vi "General Error Handler CORE.vi"(0 "[error code] (0)":i32 caption="[Fehlercode] (0)" format="%0.0f", 1 "[user-defined codes]":i32[](array[numeric]) caption="[Benutzerspezif. Codes]", 2 "[user-defined descriptions]":string[](array[string]) caption="[Benutzerspezif. Beschreibungen]", 5 "[error source] (\" \")":string caption="[Fehlerquelle] (\" \")", 7 "String to Format (not a refnum)":refnum<vi> caption="String nach Format (kein Refnum)", 9 "type of dialog (OK msg:1)":T2=enum."OK message" caption="Dialog-Typ (OK msg:1)", 11 "error in (no error)":errorcluster caption="Fehler (Eingang, kein Fehler)", 12 "[exception action] (none:0)":i32(ring) caption="[Ausnahmeaktion] (none:0)" items=["Keine Ausnahme", "Bei Übereinstimmung Fehler ignorieren", "bei Übereinstimmung Fehler ausgeben"], 13 "[exception code]":i32 caption="[Ausnahmecode]" format="%0.0f", 14 "[exception source]":string caption="[Ausnahmequelle]") -> (3 "stop event propagated":bool caption="Stopereignis propagieren", 4 "error?":bool caption="Fehler?", 6 "code out":i32 caption="Code (Ausgabe)" format="%0.0f", 8 "source out":string caption="Quelle (Ausgang)", 10 "message":string=" INSTRUKTIONEN:\r\rAllgemeine Nutzung:  Bei der Benutzung von SubVIs, die die Fehler(Eingang)-/Fehler(Ausgang)- (oder Fehler-I/O-) Struktur verwenden, plazieren Sie diesen Handler dort, wo Sie den Benutzer auf aufgetretene Fehler hinweisen wollen, typischerweise geschieht dies am Ende eines I/O-Datenpfades als letzte Aktion des Programms.  Wenn der Fehlerstatus einen Fehler angibt, erzeugt der Handler eine Nachricht, die den Fehler und dessen Ursprung beschreibt.  Ist Dialogtyp = 1 (Voreinstellung), wird die Fehlermeldung angezeigt und der Benutzer kann diese lediglich bestätigen.  Ist Dialogtyp = 2, kann der Benutzer die Meldung bestätigen oder die Programm-Ausführung abbrechen; der Abbruch eines Programms mit aktiver I/O wird jedoch nicht empfohlen.  Ist der Dialogtyp = 0, wird keine Meldung angezeigt; dieser Modus wird verwendet, um Fehler programmatisch zu behandeln, aus diesem Grunde sind auch die Fehlerausgangs-Cluster mit individuellen Terminals verbunden.  \r\rAndere Nutzungsmöglichkeit:\n\r\nLokales Testen.  Um einen Fehlercode eines SubVI oder einer Funktion zu testen, die keine Fehler-I/O-Struktur beinhalten, kann deren Fehlercode und ein Quellen-String mit den lokalen Fehlercode- und Quellenstring-Eingängen verbunden werden.  Wenn der Fehlerstatus keinen Fehler anzeigt und der Fehlercode ungleich 0 ist, werden der lokale Code und der String des Fehlereingangs-Wertes ersetzt und Fehler? wird auf TRUE (FEHLER) gesetzt." caption="Meldung", 15 "error out":errorcluster caption="Fehler (Ausgang)")   [LabVIEW 2009]
doc: "Zeigt an, ob ein Fehler aufgetreten ist. Wenn ja, gibt dieses VI eine Fehlermeldung zurück und zeigt (optional) ein Dialogfenster an."
uses:
  DialogTypeEnum.ctl
  whitespace.ctl
panel:
  in  "Case Constant\n(See Context Help)":bool
  in  "prompts":T1={"Error %d occurred at %s"="Fehler %d ist bei %s aufgetreten", "Warning %d occurred at %s"="Warnung %d ist bei %s aufgetreten", "Possible reasons: %s"="<b>Mögliche Gründe:</b>\\n%s", "Error not listed"="Dieser Fehlercode ist nicht definiert. Für diesen Code wurde keine Beschreibung erstellt oder es wurde ein Wert an den Fehlercode-Eingang verbunden, der kein Fehlercode ist.", "GetCommError x%lx"="Windows GetCommError:  Der Hex-Wert dieses Codes ist <B>x%04lx</B>.\n\nBitweise interpretiert ergibt dies:\n<B>x4000</B>: Fehler in VI für seriellen Port\n<B>x0001</B>: Empfangsqueue übergelaufen oder Zeichen wurde nach EOF-Zeichen empfangen\n<B>x0002</B>: Zeichen durch Überschreiben verloren\n<B>x0004</B>: Paritätsfehler\n<B>x0008</B>: Framing-Fehler\n<B>x0010</B>: Abbruchbedingung\n<B>x0020</B>: CTS-Timeout\n<B>x0040</B>:  DSR-Timeout\n<B>x0080</B>: RLSD-Timeout\n<B>x0100</B>: Übertragungsqueue war bei Ankunft eines neuen Zeichen bereits voll\n<B>x0200</B>: Timeout für paralleles Gerät\n<B>x0400</B>: I/O-Fehler an parallelem Gerät\n<B>x0800</B>: Paralleles Gerät nicht selektiert\n<B>x1000</B>: Kein Papier im parallelen Gerät\n<B>x8000</B>: angeforderter Modus wird nicht unterstützt oder der idComDev-Parameter ist ungültig.", "Continue"="OK", "Stop"="Stopp", "an unidentified location"="Nicht identifizierte Position", "No Error"="Kein Fehler", "Help"="Warum nicht gefunden?"} caption="Aufforderung"
  # "Reinitialisieren auf Standardwerte, um Anweisungen anzuzeigen."
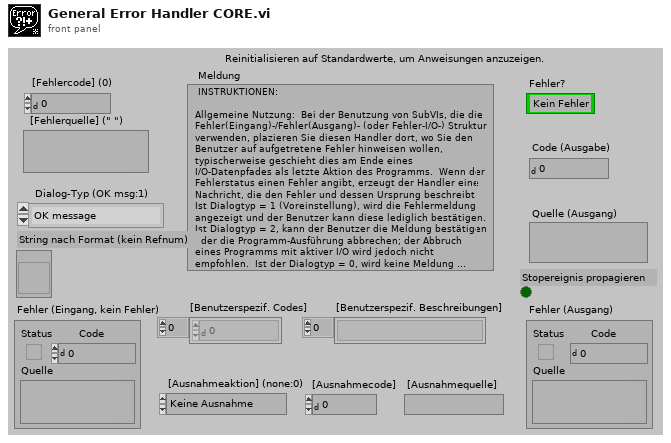
[diagram p1: front panel]
types:
  T1 = cluster{"Error %d occurred at %s":string, "Warning %d occurred at %s":string, "Possible reasons: %s":string, "Error not listed":string, "GetCommError x%lx":string, "Continue":string, "Stop":string, "an unidentified location":string, "No Error":string, "Help":string}
  T2 = typedef "DialogTypeEnum.ctl" = enum16{"no dialog", "OK message", "continue or stop message", "auto error handling dialog", "OK message + warnings", "continue/stop + warnings"}
  T3 = enum32{"invalid app kind", "Development System", "Run Time System", "Student Edition", "Embedded LabVIEW"}
  T4 = typedef "TagReturnType.ctl" = enum16{"No Tag", "<err>", "<append>"}
  T5 = typedef "whitespace.ctl" = u16
  T6 = enum32{"invalid app kind", "Development System", "Run Time System", "Student Edition", "Embedded LabVIEW", "Evaluation", "Custom"}
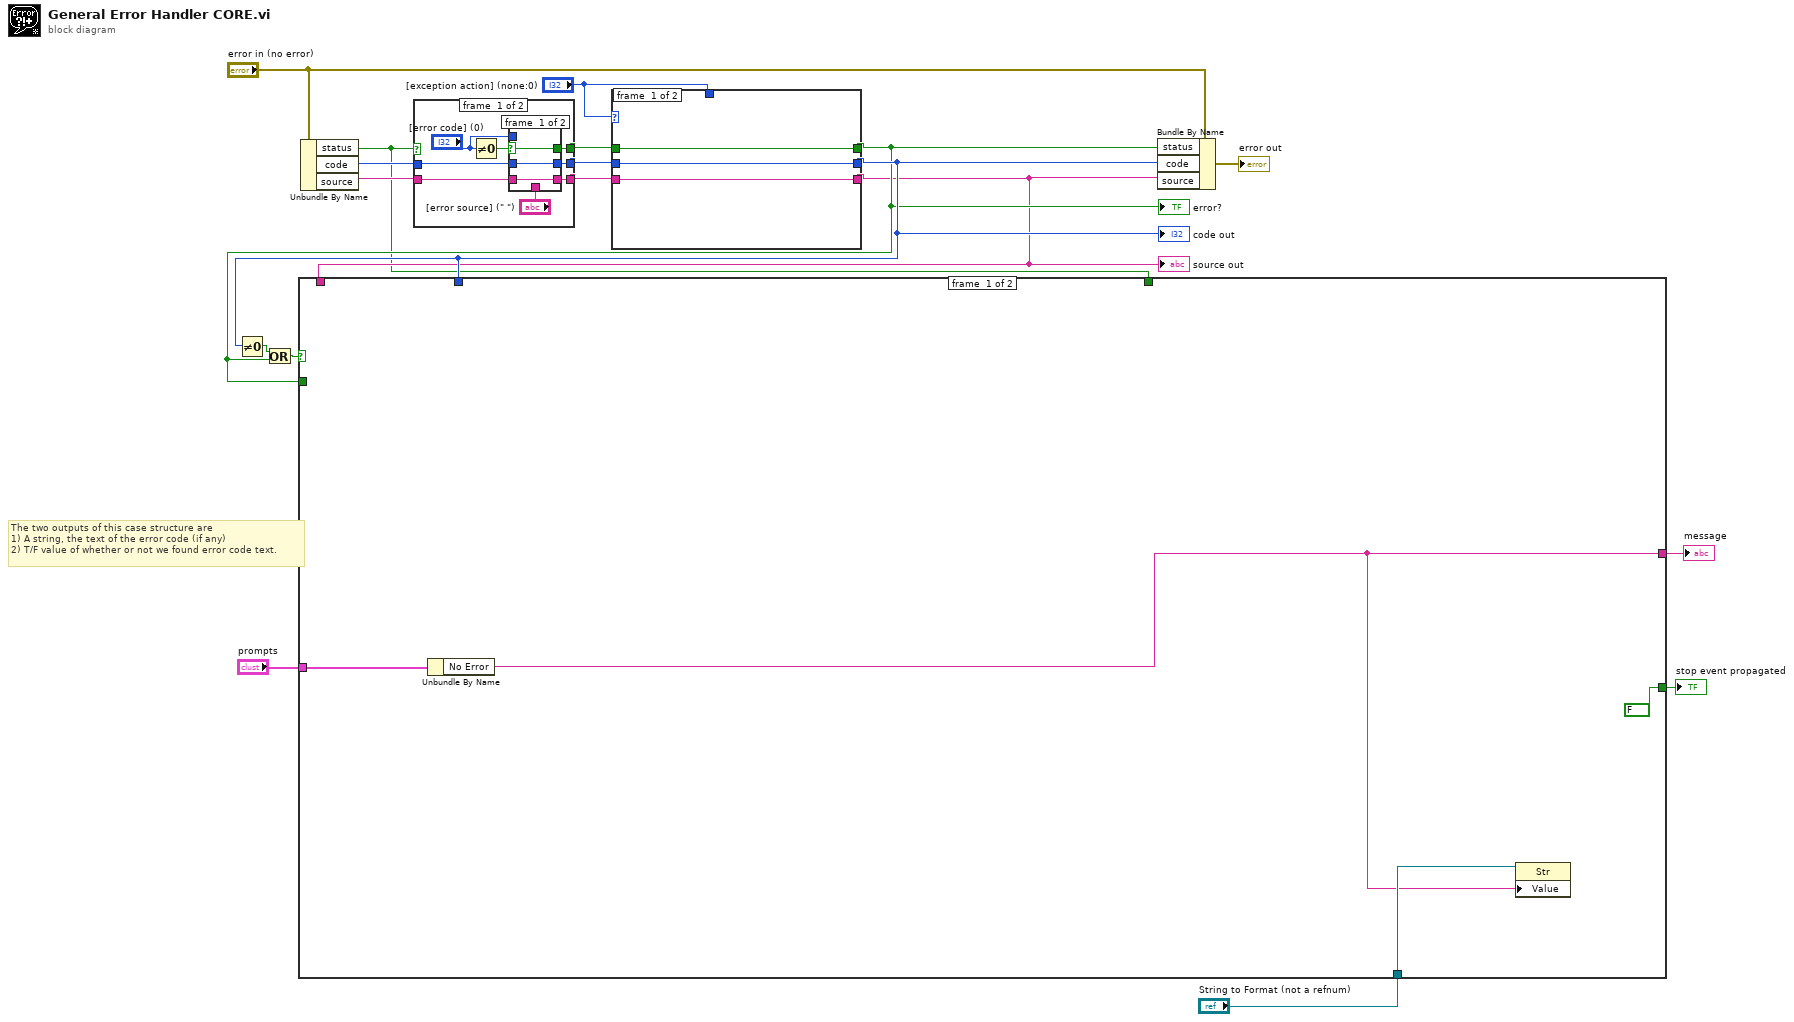
[diagram p0: block diagram]
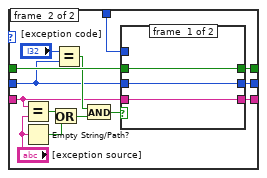
[diagram p2: hidden frame]
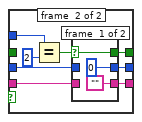
[diagram p3: hidden frame]
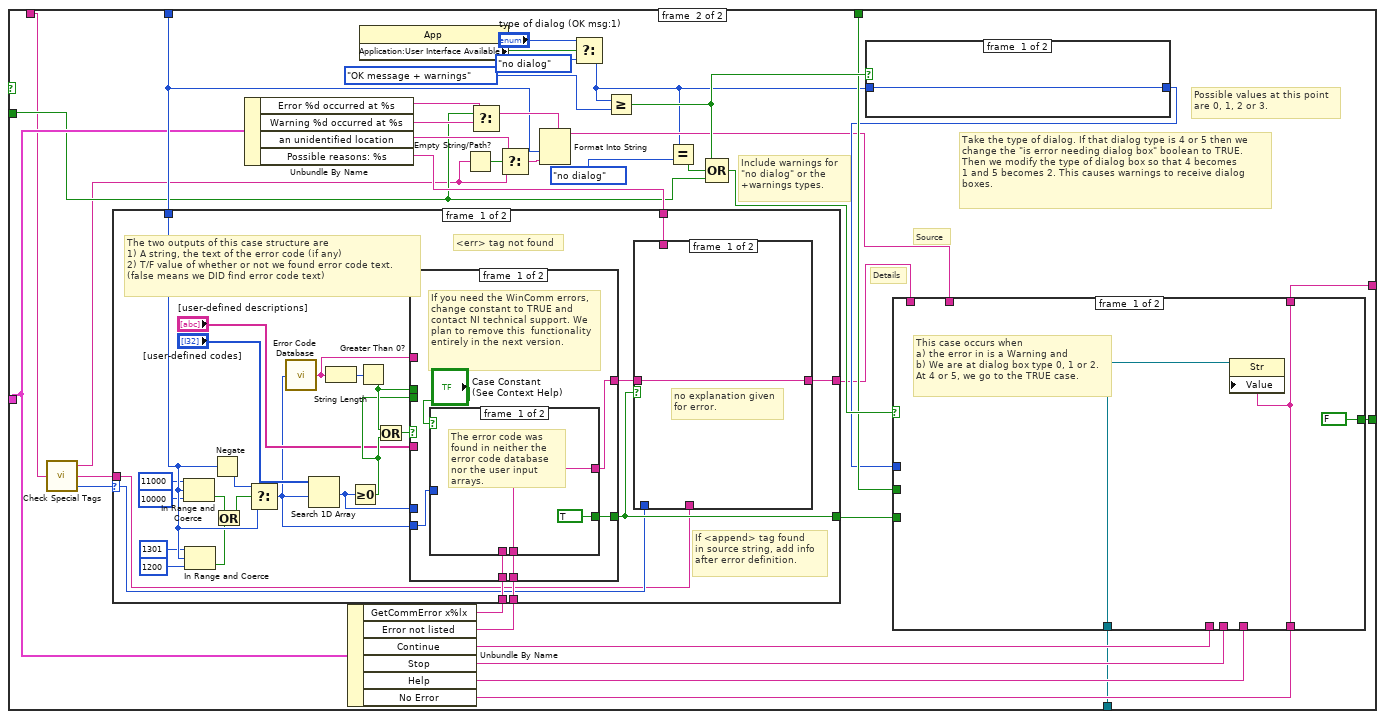
[diagram p7: hidden frame]
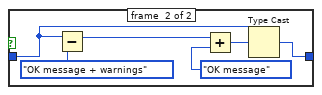
[diagram p8: hidden frame]
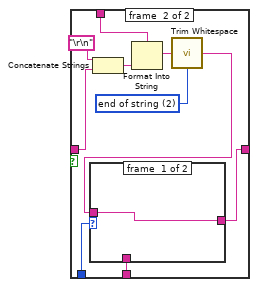
[diagram p9: hidden frame]
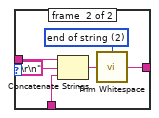
[diagram p10: hidden frame]
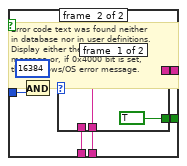
[diagram p11: hidden frame]
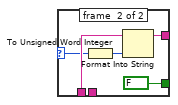
[diagram p12: hidden frame]
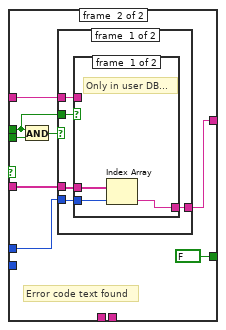
[diagram p13: hidden frame]
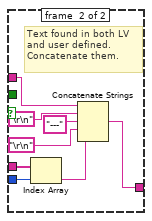
[diagram p15: hidden frame]
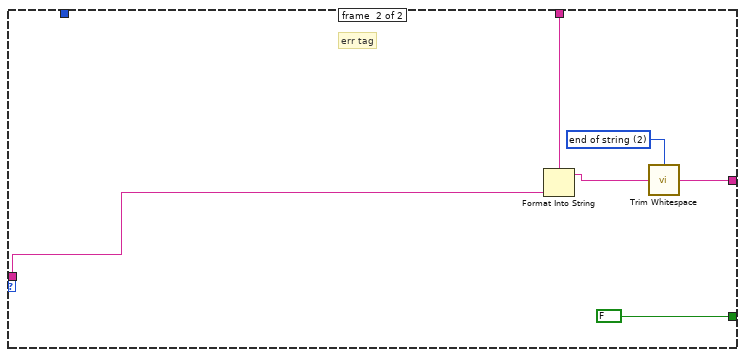
[diagram p16: hidden frame]
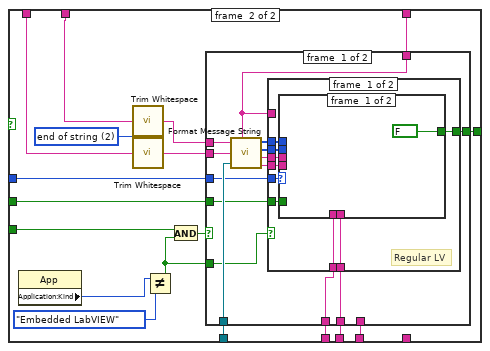
[diagram p17: hidden frame]
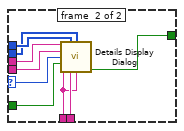
[diagram p18: hidden frame]
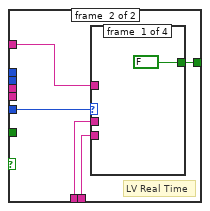
[diagram p19: hidden frame]
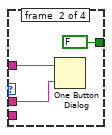
[diagram p20: hidden frame]
diagram:
  # "The two outputs of this case structure are\n1) A string, the text of the error code (if any)\n2) T/F value of whether or not we found error code text."
  n1 = Unbundle By Name("error in (no error)") -> ("status"=w3:bool, "code"=w13:i32, "source"=w17:string)
  n2 = case shown="False" w3 {
    selector: w3 -> [_ w35]
    tunnel: [w23 w34] -> w15
    tunnel: [w25 w35] -> w14
    tunnel: w13 -> [w19 w34]
    tunnel: [w21 w33] -> w16
    tunnel: w17 -> [w20 w33]
    frame #0 {
      n3 = Not Equal To 0?(x="[error code] (0)") -> (x != 0?=w26:bool)
      n4 = case shown="True" w26 {
        selector: w26 -> [w29 w32]
        tunnel: [w29 w32] -> w25
        tunnel: "[error code] (0)" -> [_ w31]
        tunnel: [w27 w31] -> w23
        tunnel: "[error source] (\" \")" -> [_ w30]
        tunnel: [w28 w30] -> w21
        tunnel: w20 -> [w28 _]
        tunnel: w19 -> [w27 _]
        frame #0 {
        }
        frame #1 {
        }
      }
    }
    frame #1 {
    }
  }
  n5 = case shown="1.." "[exception action] (none:0)" {
    tunnel: [w38 w52] -> w8
    tunnel: w14 -> [w38 w50]
    tunnel: [w37 w51] -> w11
    tunnel: w15 -> [w37 w44]
    tunnel: [w36 w41] -> w7
    tunnel: w16 -> [w36 w39]
    tunnel: "[exception action] (none:0)" -> [_ w40]
    frame #0 {
    }
    frame #1 {
      n6 = Equal?(x=w39, y="[exception source]") -> (x = y?=w46:bool)
      n7 = Empty String/Path?(string/path="[exception source]") -> (empty?=w47:bool)
      n8 = Or(x=w46, y=w47) -> (x .or. y?=w48:bool)
      n9 = Equal?(x="[exception code]", y=w44) -> (x = y?=w49:bool)
      n10 = And(x=w49, y=w48) -> (x .and. y?=w42:bool)
      n11 = case shown="True" w42 {
        tunnel: [w55 w56] -> w52
        tunnel: [w54 w60] -> w51
        tunnel: w50 -> [w55 _]
        tunnel: w44 -> [w54 w59]
        tunnel: w40 -> [_ w63]
        tunnel: [w53 w58] -> w41
        tunnel: w39 -> [w53 w57]
        frame #0 {
        }
        frame #1 {
          n12 = Equal?(x=w63, y=2) -> (x = y?=w61:bool)
          n13 = case shown="False" w61 {
            selector: w61 -> [w66 w69]
            tunnel: [0 w68] -> w60
            tunnel: w59 -> [_ w68]
            tunnel: ["" w67] -> w58
            tunnel: w57 -> [_ w67]
            tunnel: [w66 w69] -> w56
            frame #0 {
            }
            frame #1 {
            }
          }
        }
      }
    }
  }
  "source out" <- w7
  "error?" <- w8
  "code out" <- w11
  n14 = Not Equal To 0?(x=w11) -> (x != 0?=w10:bool)
  n15 = Or(x=w10, y=w8) -> (x .or. y?=w9:bool)
  n16 = case shown="True" w9 {
    tunnel: [w70 w88] -> w18
    tunnel: w11 -> [_ w103]
    tunnel: w8 -> [_ w83]
    tunnel: w7 -> [_ w75]
    tunnel: "prompts" -> [w73 w98]
    tunnel: w3 -> [_ w92]
    tunnel: [FALSE ("Stop 2") w91] -> w2
    tunnel: "String to Format (not a refnum)" -> [w71 w84]
    frame #0 {
      n17 = Unbundle By Name(w73) -> ("No Error"=w70:string)
      n18 = property class="Str"(reference=w71, "Value"=w70) -> ()  [unwired: 1 in, 2 out]
    }
    frame #1 {
      # "Include warnings for\n\"no dialog\" or the \n+warnings types."
      # "Details"
      # "Source"
      # "Possible values at this point\nare 0, 1, 2 or 3."
      # "Take the type of dialog. If that dialog type is 4 or 5 then we\nchange the \"is error needing dialog box\" boolean to TRUE.\nThen we modify the type of dialog box so that 4 becomes\n1 and 5 becomes 2. This causes warnings to receive dialog\nboxes."
      n19 = call "Check Special Tags.vi"("source"=w75) -> ("Before Tag (source)"=w74:string, "After Tag (special data)"=w108:string, "Tag Found?"=w93:T4)
      n20 = Unbundle By Name(w98) -> ("Error %d occurred at %s"=w109:string, "Warning %d occurred at %s"=w107:string, "an unidentified location"=w104:string, "Possible reasons: %s"=w90:string)
      n21 = Unbundle By Name(w98) -> ("GetCommError x%lx"=w101:string, "Error not listed"=w102:string, "Continue"=w100:string, "Stop"=w99:string, "Help"=w96:string, "No Error"=w85:string)
      n22 = case shown="\"No Tag\", \"<append>\", Default" w93 {
        selector: w93 -> [w121 _]
        tunnel: [w119 w212] -> w87
        tunnel: w103 -> [w143 _]
        tunnel: w108 -> [w120 w211]
        tunnel: w101 -> [w142 _]
        tunnel: w102 -> [w141 _]
        tunnel: [w122 FALSE] -> w97
        tunnel: w90 -> [w124 w210]
        frame #0 {
          # "If <append> tag found\nin source string, add info\nafter error definition."
          # "<err> tag not found"
          # "The two outputs of this case structure are\n1) A string, the text of the error code (if any)\n2) T/F value of whether or not we found error code text.\n(false means we DID find error code text)"
          n23 = In Range and Coerce(upper limit=11000, x=w143, lower limit=10000) -> (In Range?=w134:bool)  [unwired: 1 out]
          n24 = In Range and Coerce(upper limit=1301, x=w143, lower limit=1200) -> (In Range?=w135:bool)  [unwired: 1 out]
          n25 = Negate(x=w143) -> (-x=w137:i32)
          n26 = Or(x=w134, y=w135) -> (x .or. y?=w133:bool)
          n27 = Select(t=w137, s=w133, f=w143) -> (s? t:f=w118:i32)
          n28 = call "Error Code Database.vi"("Error Code"=w118) -> ("Error Text"=w125:string)
          n29 = Search 1D Array(1D array="[user-defined codes]", element=w118) -> (index of element=w140:i32)  [unwired: 1 in]
          n30 = String Length(string=w125) -> (length=w130:i32)
          n31 = Greater Or Equal To 0?(x=w140) -> (x >= 0?=w127:bool)
          n32 = Greater Than 0?(x=w130) -> (x > 0?=w128:bool)
          n33 = Or(x=w128, y=w127) -> (x .or. y?=w129:bool)
          n34 = case shown="False" w129 {
            tunnel: w140 -> [_ w187]
            tunnel: [w167 w185] -> w123
            tunnel: w118 -> [w163 _]
            tunnel: w142 -> [w166 _]
            tunnel: w141 -> [w165 _]
            tunnel: [w164 FALSE] -> w122
            tunnel: w128 -> [_ w184]
            tunnel: w127 -> [_ w189]
            tunnel: "[user-defined descriptions]" -> [_ w188]
            tunnel: w125 -> [_ w186]
            frame #0 {
              # "If you need the WinComm errors, change constant to TRUE and contact NI technical support. We plan to remove this  functionality entirely in the next version."
              n35 = case shown="False" "Case Constant\n(See Context Help)" {
                tunnel: [w169 w176] -> w167
                tunnel: w166 -> [_ w173]
                tunnel: w165 -> [w169 w172]
                tunnel: [TRUE w171] -> w164
                tunnel: w163 -> [_ w170]
                frame #0 {
                  # "The error code was found in neither the error code database nor the user input arrays."
                }
                frame #1 {
                  # "Error code text was found neither\nin database nor in user definitions.\nDisplay either the \"not found\" \nmessage or, if 0x4000 bit is set,\nthe windows/OS error message."
                  n36 = And(x=16384, y=w170) -> (x .and. y?=w174:i32)
                  n37 = case shown="..0" w174 {
                    selector: w174 -> [_ w179]
                    tunnel: [w178 w182] -> w176
                    tunnel: w173 -> [_ w183]
                    tunnel: w172 -> [w178 _]
                    tunnel: [TRUE FALSE] -> w171
                    frame #0 {
                    }
                    frame #1 {
                      n38 = To Unsigned Word Integer(number=w179) -> (unsigned 16bit integer=w181:u16)
                      n39 = Format Into String(format string=w183, w181) -> (resulting string=w182:string)  [unwired: 2 in, 1 out]
                    }
                  }
                }
              }
            }
            frame #1 {
              # "Error code text found"
              n40 = And(x=w184, y=w189) -> (x .and. y?=w190:bool)
              n41 = case shown="True" w190 {
                tunnel: w188 -> [w193 w208]
                tunnel: w187 -> [w192 w207]
                tunnel: w186 -> [w194 w201]
                tunnel: [w195 w205] -> w185
                tunnel: w184 -> [w196 _]
                frame #0 {
                  n42 = case shown="True" w196 {
                    tunnel: [w197 w200] -> w195
                    tunnel: w194 -> [_ w200]
                    tunnel: w193 -> [w199 _]
                    tunnel: w192 -> [w198 _]
                    frame #0 {
                      # "Only in user DB..."
                      n43 = Index Array(array=w199, index=w198) -> (element=w197:string)
                    }
                    frame #1 {
                      # "Only in LV DB..."
                    }
                  }
                }
                frame #1 {
                  # "Text found in both LV\nand user defined. \nConcatenate them."
                  n44 = Index Array(array=w208, index=w207) -> (element=w206:string)
                  n45 = Concatenate Strings(w201, "\r\n", "---" ("string"), "\r\n", w206) -> (w205:string)
                }
              }
            }
          }
          n46 = case shown="False" w122 {
            tunnel: w124 -> [_ w154]
            tunnel: [w144 w146] -> w119
            tunnel: w123 -> [w144 w151]
            tunnel: w121 -> [_ w148]
            tunnel: w120 -> [_ w147]
            frame #0 {
              # "no explanation given\nfor error."
            }
            frame #1 {
              w145 = T5 2 items=["both", "start of string", "end of string"] ("location (both)")
              n47 = Concatenate Strings("\r\n", w151) -> (w152:string)
              n48 = Format Into String(format string=w154, w152) -> (resulting string=w153:string)  [unwired: 2 in, 1 out]
              n49 = call "Trim Whitespace.vi"("string"=w153, "location (both)"=w145) -> ("trimmed string"=w149:string)
              n50 = case shown="\"<append>\"" w148 {
                tunnel: w149 -> [w155 w160]
                tunnel: [w155 w157] -> w146
                tunnel: w147 -> [_ w159]
                frame #0 {
                }
                frame #1 {
                  w156 = T5 2 items=["both", "start of string", "end of string"] ("location (both)")
                  n51 = Concatenate Strings(w160, "\r\n", w159) -> (w158:string)
                  n52 = call "Trim Whitespace.vi"("string"=w158, "location (both)"=w156) -> ("trimmed string"=w157:string)
                }
              }
            }
          }
        }
        frame #1 {
          w209 = T5 2 items=["both", "start of string", "end of string"] ("location (both)")
          # "err tag"
          n53 = Format Into String(format string=w210, w211) -> (resulting string=w213:string)  [unwired: 2 in, 1 out]
          n54 = call "Trim Whitespace.vi"("string"=w213, "location (both)"=w209) -> ("trimmed string"=w212:string)
        }
      }
      n55 = property class="App"() -> ("Application:User Interface Available"=w76:bool)  [unwired: 2 in, 2 out]
      n56 = Empty String/Path?(string/path=w74) -> (empty?=w110:bool)
      n57 = Select(t=w109, s=w83, f=w107) -> (s? t:f=w106:string)
      n58 = Select(t=w104, s=w110, f=w74) -> (s? t:f=w105:string)
      n59 = Format Into String(format string=w106, w103, w105) -> (resulting string=w86:string)  [unwired: 2 in, 1 out]
      n60 = Select(t="type of dialog (OK msg:1)", s=w76, f=DialogTypeEnum."no dialog" ("type of dialog (OK msg:1)")) -> (s? t:f=w78:T2)
      n61 = Greater Or Equal?(x=w78, y=DialogTypeEnum."OK message + warnings" ("type of dialog (OK msg:1)")) -> (x >= y?=w94:bool)
      n62 = Equal?(x=w78, y=DialogTypeEnum."no dialog" ("type of dialog (OK msg:1)")) -> (x = y?=w82:bool)
      n63 = Compound Arithmetic op=OR(w94, w82, w83) -> (w95:bool)
      n64 = case shown="True" w94 {
        tunnel: w78 -> [w111 w112]
        tunnel: [w111 w114] -> w89
        frame #0 {
        }
        frame #1 {
          n65 = Subtract(x=w112, y=DialogTypeEnum."OK message + warnings" ("type of dialog (OK msg:1)")) -> (x-y=w117:u16)
          n66 = Add(x=w117, y=DialogTypeEnum."OK message" ("type of dialog (OK msg:1)")) -> (x+y=w113:u16)
          n67 = Type Cast(type=w112, x=w113) -> (*(type *) &x=w114:T2)
        }
      }
      n68 = case shown="True" w95 {
        tunnel: w89 -> [_ w235]
        tunnel: w100 -> [_ w234]
        tunnel: w99 -> [_ w233]
        tunnel: w97 -> [_ w227]
        tunnel: w96 -> [_ w232]
        tunnel: w86 -> [_ w224]
        tunnel: w87 -> [_ w225]
        tunnel: w92 -> [_ w231]
        tunnel: [FALSE ("Stop 2") w230] -> w91
        tunnel: [w216 w229] -> w88
        tunnel: w85 -> [w216 _]
        tunnel: w84 -> [w215 w228]
        frame #0 {
          # "This case occurs when\na) the error in is a Warning and\nb) We are at dialog box type 0, 1 or 2.\nAt 4 or 5, we go to the TRUE case."
          n69 = property on="Property Node" class="Str"(reference=w215, "Value"=w216) -> ()  [unwired: 1 in, 2 out]
        }
        frame #1 {
          w218 = T5 2 items=["both", "start of string", "end of string"] ("location (both)")
          n70 = property class="App"() -> ("Application:Kind"=w221:T6)  [unwired: 2 in, 2 out]
          n71 = call "Trim Whitespace.vi"("string"=w224, "location (both)"=w218) -> ("trimmed string"=w223:string)
          n72 = call "Trim Whitespace.vi"("string"=w225, "location (both)"=w218) -> ("trimmed string"=w226:string)
          n73 = Not Equal?(x=w221, y=T3."Embedded LabVIEW" ("Application:Kind")) -> (x != y?=w219:bool)
          n74 = And(x=w227, y=w219) -> (x .and. y?=w220:bool)
          n75 = case shown="False" w220 {
            tunnel: w226 -> [w248 w289]
            tunnel: w232 -> [_ w298]
            tunnel: w234 -> [w244 w296]
            tunnel: w233 -> [w243 w295]
            tunnel: w235 -> [w246 w297]
            tunnel: [w245 w294] -> w230
            tunnel: w223 -> [w249 w290]
            tunnel: w231 -> [w242 _]
            tunnel: [w236 w291] -> w229
            tunnel: w228 -> [w247 w293]
            tunnel: w219 -> [w237 _]
            frame #0 {
              n76 = call "Format Message String.vi"("Source"=w249, "Details"=w248, "String to Format (not a refnum)"=w247) -> ("message"=w236:string, "Bold Start"=w241:i32[], "Bold Length"=w240:i32[], "Source Out"=w239:string, "Details Out"=w238:string)  [unwired: 1 in]
              n77 = case shown="True" w237 {
                tunnel: w246 -> [w258 w273]
                tunnel: [w257 w272] -> w245
                tunnel: w244 -> [w256 w271]
                tunnel: w243 -> [w255 w270]
                tunnel: w242 -> [w254 _]
                tunnel: w241 -> [w253 _]
                tunnel: w240 -> [w252 _]
                tunnel: w239 -> [w251 _]
                tunnel: w238 -> [w250 _]
                tunnel: w236 -> [_ w269]
                frame #0 {
                  # "Regular LV"
                  n78 = case shown="\"OK message\", Default" w258 {
                    selector: w258 -> [_ w265]
                    tunnel: [FALSE ("stop event propagated") w268] -> w257
                    tunnel: w256 -> [_ w266]
                    tunnel: w255 -> [_ w267]
                    tunnel: w254 -> [_ w264]
                    tunnel: w253 -> [_ w263]
                    tunnel: w252 -> [_ w262]
                    tunnel: w251 -> [_ w261]
                    tunnel: w250 -> [_ w260]
                    frame #0 {
                    }
                    frame #1 {
                      n79 = call "Details Display Dialog.vi"("Source"=w261, "Start"=w263, "Length"=w262, "Details"=w260, "dialog type"=w265, "Error or Warning"=w264, "contname"=w266, "stopname"=w267, "okname"=w266) -> ("stop event propagated"=w268:bool)  [unwired: 6 in]
                    }
                  }
                }
                frame #1 {
                  # "LV Real Time"
                  n80 = case shown="\"continue or stop message\", \"continue/stop + warnings\"" w273 {
                    tunnel: [FALSE ("stop event propagated") FALSE ("stop event propagated") FALSE ("stop event propagated") w284] -> w272
                    tunnel: w269 -> [_ w276 w283 w288]
                    tunnel: w271 -> [_ w275 w282 w287]
                    tunnel: w270 -> [_ _ w281 w286]
                    frame #0 {
                    }
                    frame #1 {
                      n81 = One Button Dialog(message=w276, button name ("OK")=w275) -> ()  [unwired: 1 out]
                    }
                    frame #2 {
                      n82 = Two Button Dialog(message=w283, 1:w281, 2:w282) -> (T button?=w279:bool)
                      n83 = Not(x=w279) -> (.not. x?=w278:bool)
                      n84 = Stop(stop? (T)=w278) -> ()
                    }
                    frame #3 {
                      n85 = Two Button Dialog(message=w288, 1:w286, 2:w287) -> (T button?=w285:bool)
                      n86 = Not(x=w285) -> (.not. x?=w284:bool)
                    }
                  }
                }
              }
            }
            frame #1 {
              w292 = "\r\n"
              n87 = Concatenate Strings(w290, w292, w292, w289) -> (w291:string)
              n88 = call "Not Found Dialog.vi"("Help"=w298, "Message"=w291, "Stop"=w295, "Continue"=w296, "type of dialog (OK msg:1)"=w297) -> ("stop event propagated"=w294:bool)  [unwired: 1 in]
              n89 = property on="Property Node" class="Str"(reference=w293, "Value"=w291) -> ()  [unwired: 1 in, 2 out]
            }
          }
        }
      }
    }
  }
  "message" <- w18
  "stop event propagated" <- w2
  n90 = Bundle By Name(cluster="error in (no error)", "status"=w8, "code"=w11, "source"=w7) -> (→"error out":errorcluster)
